vi "MQTT_PubRec_Read.vi"(8 "error in (no error)":errorcluster, 11 "connection ID":refnum<k5>) -> (0 "error out":errorcluster, 2 "Message ID":u16=10 format="%x", 3 "connection ID out":refnum<k5>)   [LabVIEW 2018, in "MQTT_Functions.lvlib"]
doc: "© 2015 - daq.io, LLC - Peter Adelhardt"
uses:
  MQTT_Functions.lvlib
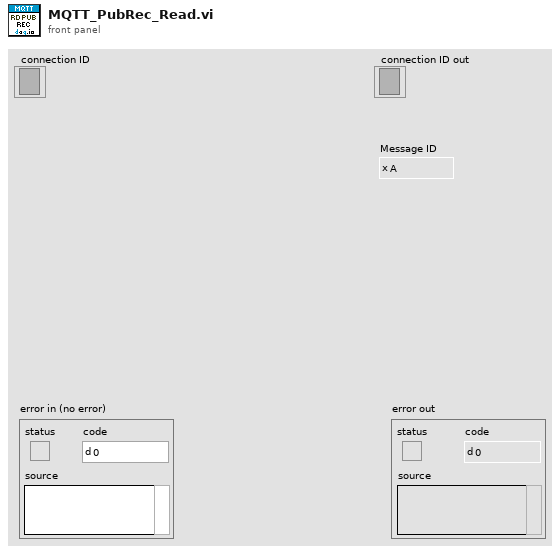
[diagram p1: front panel]
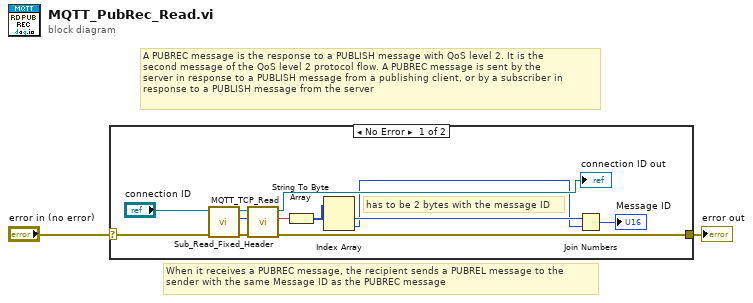
[diagram p0: block diagram]
diagram:
  # "When it receives a PUBREC message, the recipient sends a PUBREL message to the\nsender with the same Message ID as the PUBREC message"
  # "A PUBREC message is the response to a PUBLISH message with QoS level 2. It is the\nsecond message of the QoS level 2 protocol flow. A PUBREC message is sent by the\nserver in response to a PUBLISH message from a publishing client, or by a subscriber in\nresponse to a PUBLISH message from the server"
  n1 = case shown="No Error" "error in (no error)" {
    selector: "error in (no error)" -> [w11 w15]
    tunnel: [w5 w15] -> w1
    frame No Error {
      # "has to be 2 bytes with the message ID"
      n2 = call "Sub_Read_Fixed_Header.vi"("error in (no error)"=w11, "connection ID"="connection ID") -> ("error out"=w6:errorcluster, "Remaining Length"=w12:u32, "connection ID out"=w3:refnum<k5>)  [unwired: 3 in, 4 out]
      n3 = call "MQTT_TCP_Read.vi"("error in (no error)"=w6, "bytes to read"=w12, "connection ID"=w3) -> ("error out"=w5:errorcluster, "data out"=w7:string, "connection ID out"=→"connection ID out":refnum<k5>)  [unwired: 6 in]
      n4 = String To Byte Array(string=w7) -> (unsigned byte array=w8:u8[])
      n5 = Index Array(array=w8) -> (element #1=w10:u8, element #2=w9:u8)  [unwired: 2 in]
      n6 = Join Numbers(hi=w10, lo=w9) -> ((hi.lo)=→"Message ID":u16)
    }
    frame Error {
    }
  }
  "error out" <- w1
